vi "Nontarget.vi"(10 "Target_Total":path=path "C:/Users/Jaehong/Desktop/Classifiers/data/통합LDAs/kang/target_order.txt", 11 "Mius_flash_order":path=path "C:/Users/Jaehong/Desktop/Classifiers/data/통합LDAs/kang/target_order.txt") -> (3 "Nontarget_order":i64[](array[numeric]))   [LabVIEW 2014]
uses:
  <vilib>/Utility/file.llb/Read From Spreadsheet File (I64).vi
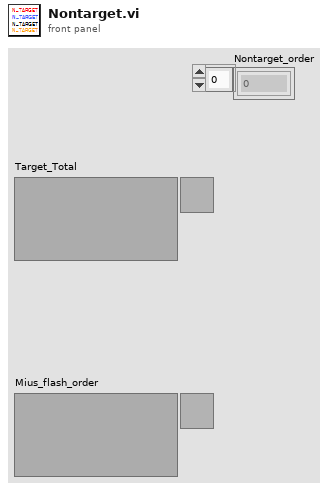
[diagram p1: front panel]
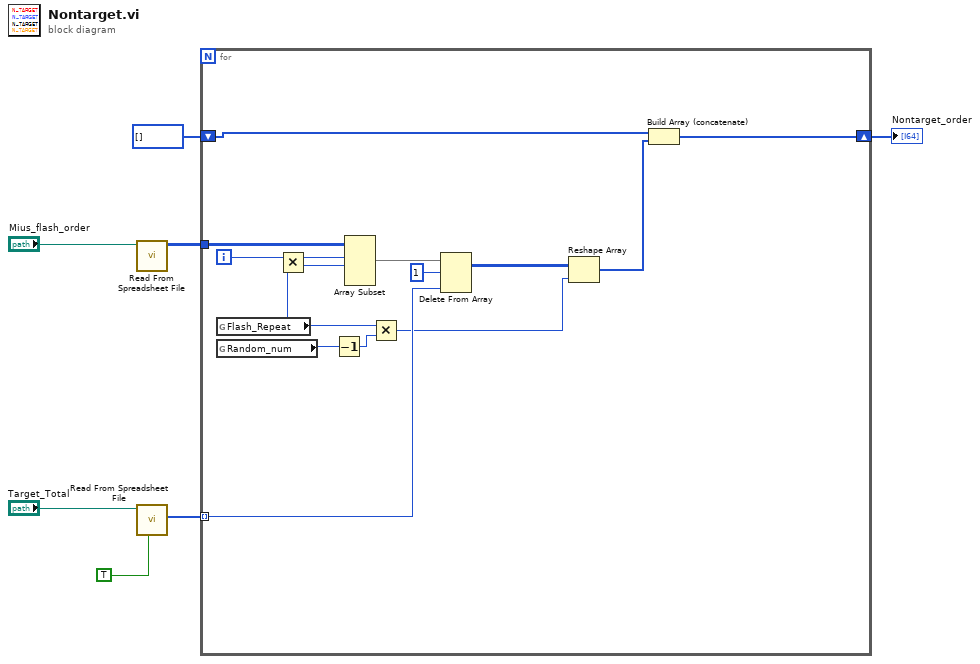
[diagram p0: block diagram]
diagram:
  n1 = call-poly <vilib>:"Read From Spreadsheet File.vi"("file path (dialog if empty)"="Mius_flash_order") -> ("all rows"=w4:i64[][])  [unwired: 6 in, 4 out]
  n2 = call-poly <vilib>:"Read From Spreadsheet File.vi"("transpose (no:F)"=TRUE, "file path (dialog if empty)"="Target_Total") -> ("first row"=w3:i64[])  [unwired: 5 in, 4 out]
  n3 = for {
    tunnel: w4 -> [w21]
    tunnel: w3 -> [w16] mode=indexing
    shift-right: [w9] -> w1
    shift-left: i64[] [] -> [w8]
    i -> [w20]
    n4 = global read "Control_Panel.vi" "Flash_Repeat"() -> (w12:i32)
    n5 = global read "Control_Panel.vi" "Random_num"() -> (w14:i32)
    n6 = Multiply(x=w20, y=w12) -> (x*y=w19:i32)
    n7 = Decrement(x=w14) -> (x-1=w13:i32)
    n8 = Array Subset(array=w21, index (row)=w19, length (row)=w12) -> (w18:i64[][])  [unwired: 2 in]
    n9 = Multiply(x=w12, y=w13) -> (x*y=w11:i32)
    n10 = Delete From Array(array=w18, length=1, index (col)=w16) -> (array with subset deleted=w15:i64[][])  [unwired: 1 in, 1 out]
    n11 = Reshape Array(w15, w11) -> (w10:i64[])
    n12 = Build Array (concatenate)(w8, w10) -> (w9:i64[])
  }
  "Nontarget_order" <- w1
